vi "Obtain Notifiers and Queues.vi"(8 "error in (no error)":errorcluster, 9 "Data Queue Names":string[](array[string]), 10 "Data Notifier Names":string[](array[string]), 11 "Task Base in":refnum<class "Task Base.lvclass">) -> (0 "error out":errorcluster, 3 "Task Base out":refnum<class "Task Base.lvclass">)   [LabVIEW 2023, in "HAL GOOP4.lvlib" / "Task Base.lvclass"]
uses:
  Task Base.lvclass
  Task Base.lvclass/Task Base.ctl
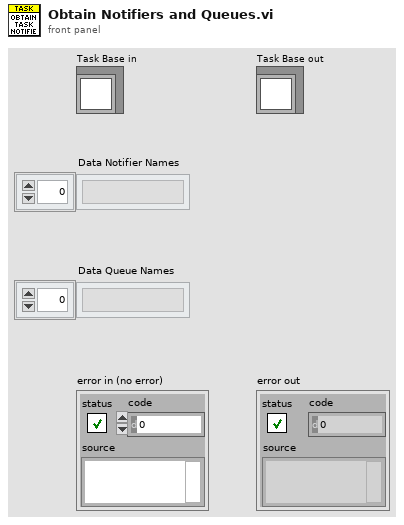
[diagram p1: front panel]
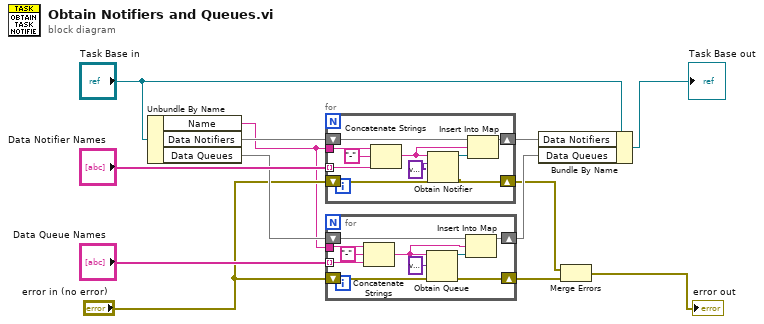
[diagram p0: block diagram]
diagram:
  n1 = Unbundle By Name("Task Base in") -> ("Name"=w8:string, "Data Notifiers"=w10:map{string, refnum<notifier>}, "Data Queues"=w11:map{string, refnum<queue>})
  n2 = for {
    tunnel: w8 -> [w22]
    tunnel: "Data Notifier Names" -> [w16] mode=indexing
    shift-right: [w21] -> w6
    shift-left: w10 -> [w23]
    shift-right: [w15] -> w3
    shift-left: "error in (no error)" -> [w14]
    n3 = Concatenate Strings(w22, "-" ("string"), w16) -> (w17:string)
    n4 = Obtain Notifier(name (unnamed)=w17, notification data type=variant ("element data type"), error in (no error)=w14) -> (notifier out=w18:refnum<notifier>, error out=w15:errorcluster)  [unwired: 1 in, 1 out]
    n5 = Insert Into Map(map in=w23, key=w17, value=w18) -> (map out=w21:map{string, refnum<notifier>})  [unwired: 2 out]
  }
  n6 = for {
    shift-right: [w30] -> w5
    shift-left: w11 -> [w31]
    tunnel: "Data Queue Names" -> [w28] mode=indexing
    tunnel: w8 -> [w27]
    shift-right: [w26] -> w4
    shift-left: "error in (no error)" -> [w25]
    n7 = Concatenate Strings(w27, "-" ("string"), w28) -> (w24:string)
    n8 = Obtain Queue(name (unnamed)=w24, element data type=variant, error in (no error)=w25) -> (queue out=w33:refnum<queue>, error out=w26:errorcluster)  [unwired: 2 in, 1 out]
    n9 = Insert Into Map(map in=w31, key=w24, value=w33) -> (map out=w30:map{string, refnum<queue>})  [unwired: 2 out]
  }
  n10 = Bundle By Name(cluster="Task Base in", "Data Notifiers"=w6, "Data Queues"=w5) -> (→"Task Base out":refnum<class "Task Base.lvclass">)
  n11 = Merge Errors(w3, w4) -> (→"error out":errorcluster)
